vi "Acquire.Image.vi"(8 "error in":errorcluster, 11 "camera.nit in":refnum<class "camera.lvclass">) -> (0 "error out":errorcluster, 2 "buffer":u16[][](array[numeric]))   [LabVIEW 2020, in "camera.lvclass"]
uses:
  camera.lvclass
  lib/O-PL.dll
panel:
  out "Intensity Graph":u16[][](graph)
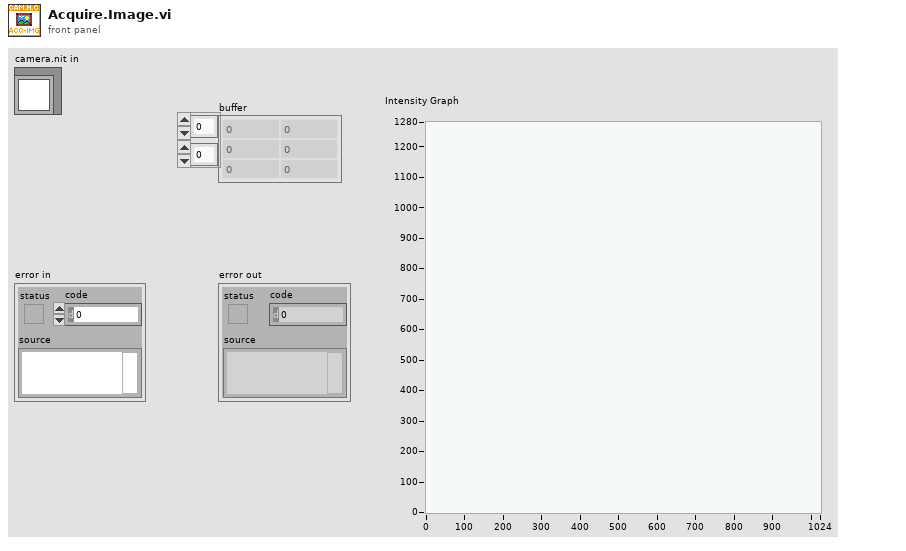
[diagram p1: front panel]
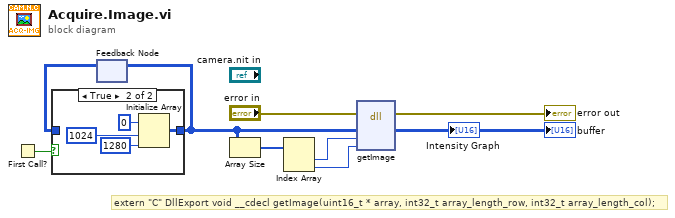
[diagram p0: block diagram]
diagram:
  # "extern \"C\" DllExport void __cdecl getImage(uint16_t * array, int32_t array_length_row, int32_t array_length_col);"
  n1 = First Call?() -> (First Call?: T/F=w9:bool)
  n2 = feedback #1() -> (w8:u16[][])  [unwired: 1 in]
  n3 = case shown="True" w9 {
    tunnel: w8 -> [w10 _]
    tunnel: [w10 w11] -> w5
    frame False {
    }
    frame True {
      n4 = Initialize Array(u16 0 ("element"), 1024 ("dimension size"), 1280 ("dimension size")) -> (w11:u16[][])
    }
  }
  n5 = feedback-in #1(w5) -> ()
  n6 = Array Size(array=w5) -> (size(s)=w7:i32[])
  n7 = Index Array(array=w7) -> (element #1=w4:i32, element #2=w6:i32)  [unwired: 2 in]
  n8 = dll-call lib="D:/UNSW - New/v0.8.3/lib/O-PL.dll" fn="getImage"(error in="error in", "array"=w5, "array_length_row"=w4, "array_length_col"=w6) -> (error out=→"error out":errorcluster, "array"=→"buffer" →"Intensity Graph":u16[][])  [unwired: 4 in, 2 out]
